vi "Full_LabviewGUI.vi"() -> ()   [LabVIEW 2022 SP3]
doc: "The UDP protocol differs from TCP in that there is no error-checking with the packets of information that are sent, and thus no guarantee whatsoever that an intended recipient will actually receive a given piece of data.\n\nUDP does offer the ability to \"broadcast\" data across a network--simply specify an IP Address of all ones (255.255.255.255) to attempt to broadcast information network-wide. Keep in mind that routers and other network hardware will generally refuse to forward the broadcast beyond certain points, so the extent of the broadcast will in practice be limited."
uses:
  <vilib>/vision/NI_Vision_Development_Module.lvlib
panel:
  out "Sensor 2 (cm)":dbl format="%#_4g"
  out "Sensor 1 (cm)":dbl format="%#_4g"
  in  "?":bool
  in  "Start Automatic Path Following":bool
  out "Image Out":T1(plugin-control)
  in  "Stop (F)":bool caption="Stop Tracking Path"
  out "XY Graph":cluster{"x":sgl, "y":sgl}[](graph)
  in  "Turn left":bool
  in  "Turn right":bool
  in  "Backward":bool
  in  "Forward":bool
  # "User Manual"
  # "1. Manual Control\nTo control the robot using manual mode, hover the cusor on the button and hold on to the click button to move the robot, stop holding the cursor will make the robot stop.\n    The Manual Control panel will be disabled and grayed out when automatic path following is running.\n\n2. Ultrasonic Sensors Data\nThe Ultrasonic Sensors Data panel shows the realtime distance from received from esp32 in the unit of cm.\n\n3. Start Automatic Path Following\nThe Start Automatic Path Following button will open up the terminal and start an anaconda kernel to run the python script that does: obstacle detection, path finding and MPC which does path following. \n    Close windows generated by the python session after its done (recommended)\n\n4. Realtime image and XY graph\nThe two panels shows the location of the robot with its track. Click on the button \"Stop Tracking Path\" to stop plotting on the graph.\n\n5. STOP\nThe stop button terminates all the process and send a final command to terminate the python kernel and stops the robot."
  # "The STOP button will terminate GUI, stop \nthe python kernel and set Jetbot speed to 0"
  # "Manual Control"
  # "Ultrasonic Sensors Data"
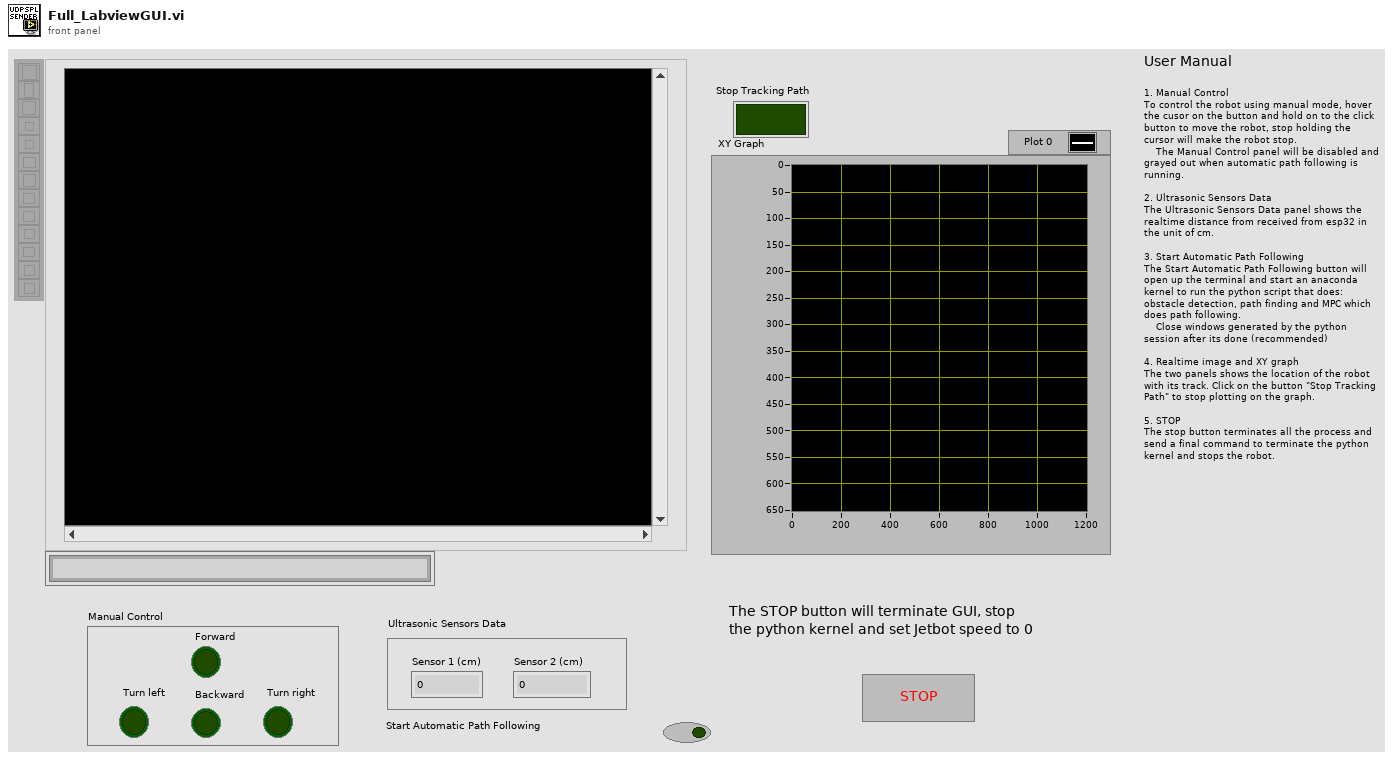
[diagram p1: front panel]
types:
  T1 = typedef "IMAQ Image.ctl" = refnum<image>
  T2 = typedef "Image Type" = u32
  T3 = enum8{"Enabled", "Disabled", "Disabled and Grayed Out"}
  T4 = cluster{"Position":cluster{"x":sgl, "y":sgl}, "Angle":sgl, "Scale":sgl, "Score":sgl, "Bounding Box":cluster{"x":sgl, "y":sgl}[]}[]
  T5 = cluster{"Matches (Pattern Matching 1)[0]":cluster{"Position":cluster{"x":sgl, "y":sgl}, "Angle":sgl, "Scale":sgl, "Score":sgl, "Bounding Box":cluster{"x":sgl, "y":sgl}[]}, "Matches (Pattern Matching 1)[1]":cluster{"Position":cluster{"x":sgl, "y":sgl}, "Angle":sgl, "Scale":sgl, "Score":sgl, "Bounding Box":cluster{"x":sgl, "y":sgl}[]}, "Matches (Pattern Matching 1)[2]":cluster{"Position":cluster{"x":sgl, "y":sgl}, "Angle":sgl, "Scale":sgl, "Score":sgl, "Bounding Box":cluster{"x":sgl, "y":sgl}[]}, "Matches (Pattern Matching 1)[3]":cluster{"Position":cluster{"x":sgl, "y":sgl}, "Angle":sgl, "Scale":sgl, "Score":sgl, "Bounding Box":cluster{"x":sgl, "y":sgl}[]}}
  T6 = cluster{"Bounding Box[0]":cluster{"x":sgl, "y":sgl}, "Bounding Box[1]":cluster{"x":sgl, "y":sgl}, "Bounding Box[2]":cluster{"x":sgl, "y":sgl}, "Bounding Box[3]":cluster{"x":sgl, "y":sgl}}
  T7 = cluster{"[0]":sgl, "[1]":sgl, "[2]":sgl, "[3]":sgl}
  T8 = cluster{"[0]":i32, "[1]":i32, "[2]":i32, "[3]":i32}
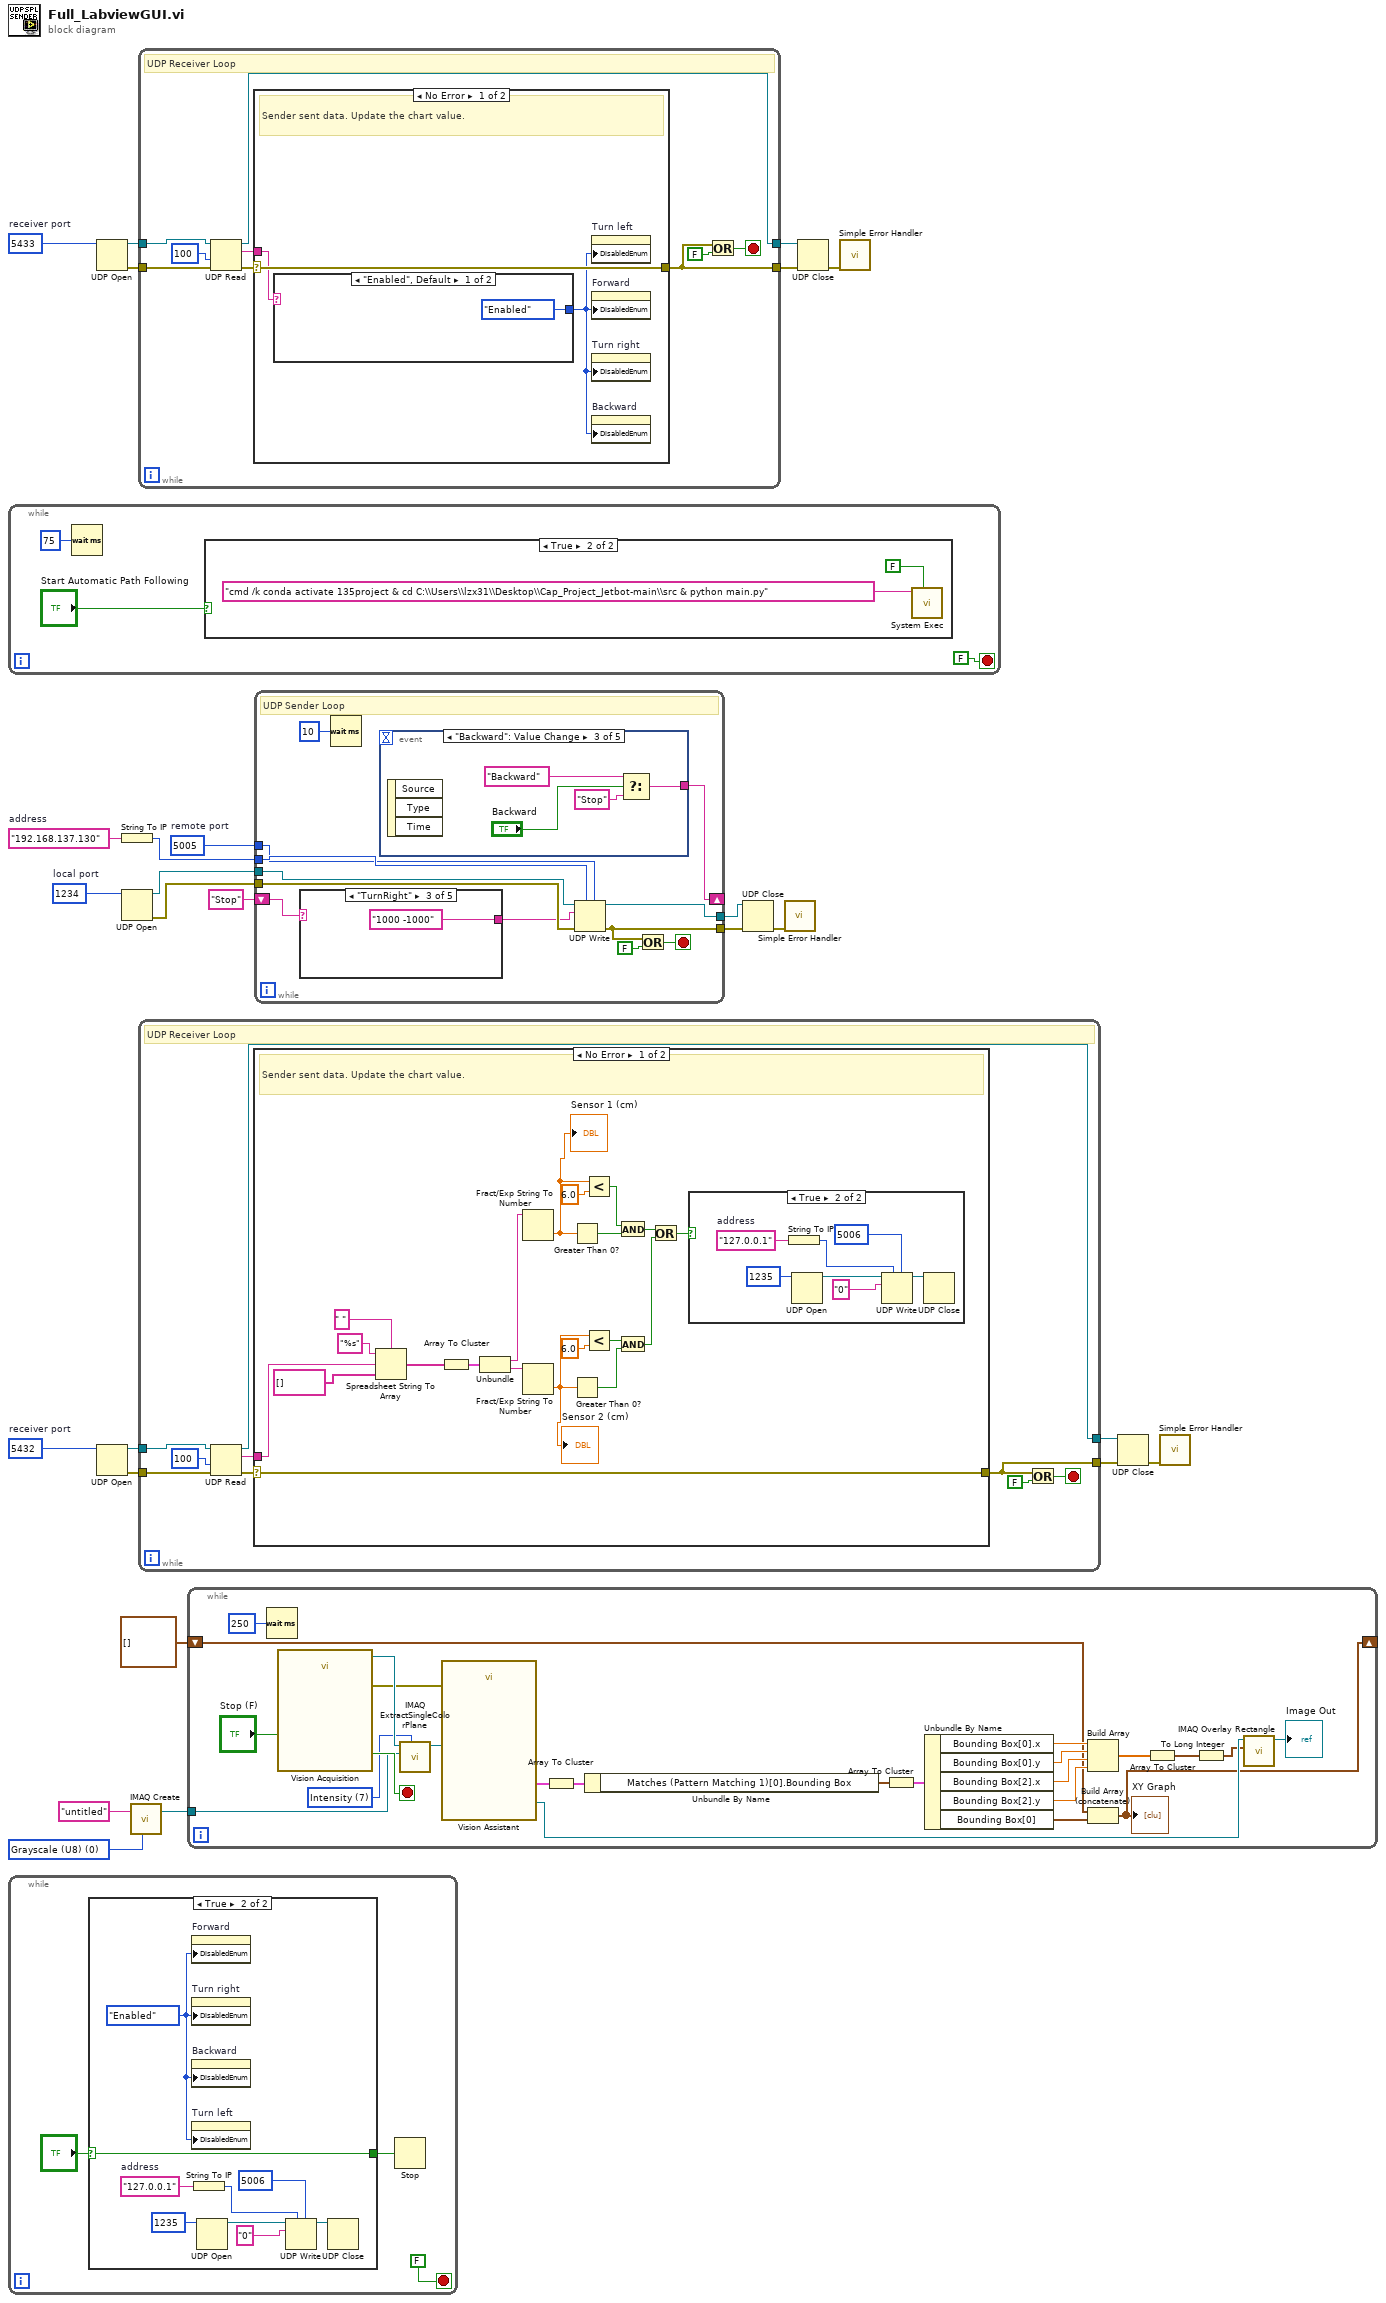
[diagram p0: block diagram]
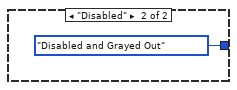
[diagram p2: hidden frame]
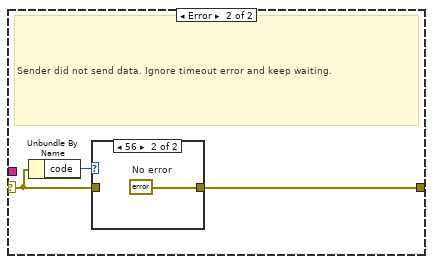
[diagram p3: hidden frame]
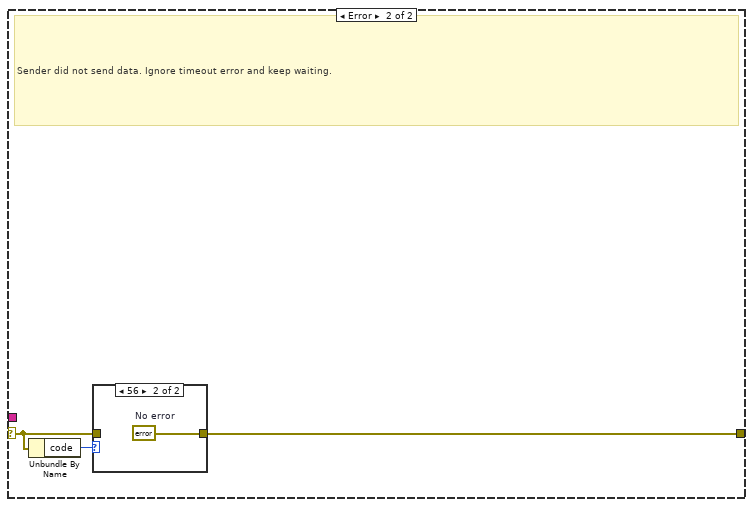
[diagram p8: hidden frame]
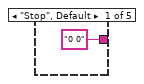
[diagram p10: hidden frame]
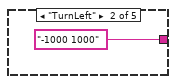
[diagram p11: hidden frame]
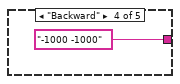
[diagram p12: hidden frame]
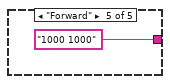
[diagram p13: hidden frame]
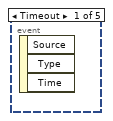
[diagram p14: hidden frame]
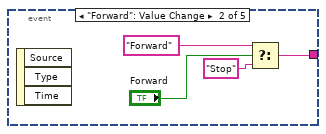
[diagram p15: hidden frame]
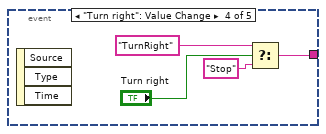
[diagram p16: hidden frame]
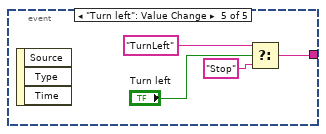
[diagram p17: hidden frame]
diagram:
  w1 = u16 5433  # receiver port
  w9 = T2 0 items=["Grayscale (U8)", "Grayscale (I16)", "Grayscale (SGL)", "Complex (CSG)", "RGB (U32)", "HSL (U32)", "RGB (U64)", "Grayscale (U16)"] ("Image Type")
  w11 = u16 5432  # receiver port
  w18 = u16 5005  # remote port
  w19 = u16 1234  # local port
  w24 = "192.168.137.130"  # address
  n1 = while {
    stop <- FALSE stop-if-true
    n2 = Wait (ms)(milliseconds to wait=u32 75) -> ()  [unwired: 1 out]
    n3 = case shown="True" "Start Automatic Path Following" {
      frame False {
      }
      frame True {
        n4 = call <vilib>:"System Exec.vi"("wait until completion? (T)"=FALSE, "command line"="cmd /k conda activate 135project & cd C:\\Users\\lzx31\\Desktop\\Cap_Project_Jetbot-main\\src & python main.py") -> ()  [unwired: 6 in, 4 out]
      }
    }
  }
  n5 = while {
    stop <- FALSE stop-if-true
    n6 = case shown="True" "?" {
      selector: "?" -> [w35 w37]
      tunnel: [w35 w37] -> w33
      frame False {
      }
      frame True {
        w36 = T3."Enabled" ("Disabled")
        w43 = "127.0.0.1"  # address
        n7 = property on="Forward" class="Bool (strict)"("DisabledEnum"=w36) -> ()  [unwired: 2 in, 2 out]
        n8 = property on="Turn right" class="Bool (strict)"("DisabledEnum"=w36) -> ()  [unwired: 2 in, 2 out]
        n9 = property on="Backward" class="Bool (strict)"("DisabledEnum"=w36) -> ()  [unwired: 2 in, 2 out]
        n10 = property on="Turn left" class="Bool (strict)"("DisabledEnum"=w36) -> ()  [unwired: 2 in, 2 out]
        n11 = String To IP(1:w43) -> (0:w42:u32)
        n12 = UDP Open(11:u16 1235 ("port")) -> (port=w41:refnum<k16>)  [unwired: 4 in, 2 out]
        n13 = UDP Write(address=w42, port or service name=u16 5006, connection ID=w41, data in="0") -> (3:w39:refnum<k16>)  [unwired: 2 in, 1 out]
        n14 = UDP Close(connection ID=w39) -> ()  [unwired: 1 in, 2 out]
      }
    }
    n15 = Stop(stop? (T)=w33) -> ()
  }
  n16 = UDP Open(11:w1) -> (port=w2:refnum<k16>, 0:w3:errorcluster)  [unwired: 4 in, 1 out]
  n17 = UDP Open(11:w11) -> (port=w12:refnum<k16>, 0:w13:errorcluster)  [unwired: 4 in, 1 out]
  n18 = String To IP(1:w24) -> (0:w22:u32)
  n19 = UDP Open(11:w19) -> (port=w21:refnum<k16>, 0:w20:errorcluster)  [unwired: 4 in, 1 out]
  n20 = call "IMAQ Create"("Image Name"="untitled", "Image Type"=w9) -> ("New Image"=w8:T1)  [unwired: 3 in, 1 out]
  n21 = while {
    tunnel: w2 -> [w53]
    tunnel: [w45] -> w6
    tunnel: w3 -> [w50]
    tunnel: [w46] -> w4
    stop <- w51 stop-if-true
    # "UDP Receiver Loop"
    n22 = UDP Read(connection ID=w53, timeout ms (25000)=100, 8:w50) -> (data out=w48:string, error out=w47:errorcluster, 3:w45:refnum<k16>)  [unwired: 3 out]
    n23 = case shown="No Error" w47 {
      selector: w47 -> [w56 w60]
      tunnel: w48 -> [w55 _]
      tunnel: [w56 w59] -> w46
      frame No Error {
        # "Sender sent data. Update the chart value."
        n24 = case shown="\"Enabled\", Default" w55 {
          tunnel: [T3."Enabled" ("Disabled") T3."Disabled and Grayed Out" ("Disabled")] -> w54
          frame "Enabled", Default {
          }
          frame "Disabled" {
          }
        }
        n25 = property on="Turn left" class="Bool (strict)"("DisabledEnum"=w54) -> ()  [unwired: 2 in, 2 out]
        n26 = property on="Forward" class="Bool (strict)"("DisabledEnum"=w54) -> ()  [unwired: 2 in, 2 out]
        n27 = property on="Turn right" class="Bool (strict)"("DisabledEnum"=w54) -> ()  [unwired: 2 in, 2 out]
        n28 = property on="Backward" class="Bool (strict)"("DisabledEnum"=w54) -> ()  [unwired: 2 in, 2 out]
      }
      frame Error {
        # "Sender did not send data. Ignore timeout error and keep waiting."
        n29 = Unbundle By Name(w60) -> ("code"=w61:i32)
        n30 = case shown="56" w61 {
          tunnel: w60 -> [w62 _]
          tunnel: [w62 w63] -> w59
          frame Default {
          }
          frame 56 {
            w63 = errorcluster {"status"=FALSE, "code"=0, "source"=""}  # No error
          }
        }
      }
    }
    n31 = Or(x=w46, y=FALSE ("Stop 2")) -> (x .or. y?=w51:bool)
  }
  n32 = while {
    tunnel: w12 -> [w72]
    tunnel: [w64] -> w16
    tunnel: w13 -> [w69]
    tunnel: [w65] -> w14
    stop <- w70 stop-if-true
    # "UDP Receiver Loop"
    n33 = UDP Read(connection ID=w72, timeout ms (25000)=100, 8:w69) -> (data out=w67:string, error out=w66:errorcluster, 3:w64:refnum<k16>)  [unwired: 3 out]
    n34 = case shown="No Error" w66 {
      selector: w66 -> [w92 w101]
      tunnel: w67 -> [w80 _]
      tunnel: [w92 w100] -> w65
      frame No Error {
        # "Sender sent data. Update the chart value."
        n35 = Spreadsheet String To Array(delimiter (Tab)=" ", format string="%s", spreadsheet string=w80, array type (2D Dbl)=string[] []) -> (array=w88:string[])
        n36 = Array To Cluster(array=w88) -> (cluster=w87:cluster{"[0]":string, "[1]":string})
        n37 = Unbundle(w87) -> ("[0]"=w76:string, "[1]"=w75:string)
        n38 = Fract/Exp String To Number(string=w76) -> (number=w74:dbl)  [unwired: 3 in, 1 out]
        "Sensor 1 (cm)" <- w74
        n39 = Fract/Exp String To Number(string=w75) -> (number=w73:dbl)  [unwired: 3 in, 1 out]
        "Sensor 2 (cm)" <- w73
        n40 = Greater Than 0?(x=w74) -> (x > 0?=w86:bool)
        n41 = Greater Than 0?(x=w73) -> (x > 0?=w84:bool)
        n42 = Less?(x=w74, y=6.0 ("x")) -> (x < y?=w85:bool)
        n43 = Less?(x=w73, y=6.0) -> (x < y?=w83:bool)
        n44 = And(x=w85, y=w86) -> (x .and. y?=w82:bool)
        n45 = And(x=w83, y=w84) -> (x .and. y?=w81:bool)
        n46 = Or(x=w82, y=w81) -> (x .or. y?=w79:bool)
        n47 = case shown="True" w79 {
          frame False {
          }
          frame True {
            w98 = "127.0.0.1"  # address
            n48 = String To IP(1:w98) -> (0:w97:u32)
            n49 = UDP Open(11:u16 1235 ("port")) -> (port=w96:refnum<k16>)  [unwired: 4 in, 2 out]
            n50 = UDP Write(address=w97, port or service name=u16 5006, connection ID=w96, data in="0") -> (3:w94:refnum<k16>)  [unwired: 2 in, 1 out]
            n51 = UDP Close(connection ID=w94) -> ()  [unwired: 1 in, 2 out]
          }
        }
      }
      frame Error {
        # "Sender did not send data. Ignore timeout error and keep waiting."
        n52 = Unbundle By Name(w101) -> ("code"=w102:i32)
        n53 = case shown="56" w102 {
          tunnel: w101 -> [w103 _]
          tunnel: [w103 w104] -> w100
          frame Default {
          }
          frame 56 {
            w104 = errorcluster {"status"=FALSE, "code"=0, "source"=""}  # No error
          }
        }
      }
    }
    n54 = Or(x=w65, y=FALSE ("Stop 2")) -> (x .or. y?=w70:bool)
  }
  n55 = while {
    tunnel: w8 -> [w126]
    shift-right: [w107] -> _
    shift-left: cluster{"x":sgl, "y":sgl}[] [] -> [w106]
    stop <- w127 stop-if-true
    w124 = 7 items=["Red", "Green", "Blue", "Hue", "Saturation", "Luminance", "Value", "Intensity"] ("Color Plane")
    n56 = Wait (ms)(milliseconds to wait=u32 250 ("millisecond timer value")) -> ()  [unwired: 1 out]
    n57 = call "Vision Acquisition"("Stop (F)"="Stop (F)") -> ("Image Out"=w125:T1, "Stopped"=w127:bool, "error out"=w122:errorcluster)  [unwired: 24 in]
    n58 = call "IMAQ ExtractSingleColorPlane"("Color Plane"=w124, "Image Dst"=w126, "Image Src"=w125) -> ("Image Dst Out"=w123:T1)  [unwired: 7 in, 1 out]
    n59 = call "Vision Assistant"("Image In"=w123, "error in"=w122) -> ("Image Out"=w113:T1, "Matches (Pattern Matching 1)"=w121:T4)  [unwired: 23 in, 1 out]
    n60 = Array To Cluster(array=w121) -> (cluster=w120:T5)
    n61 = Unbundle By Name(w120) -> ("Matches (Pattern Matching 1)[0].Bounding Box"=w119:cluster{"x":sgl, "y":sgl}[])
    n62 = Array To Cluster(array=w119) -> (cluster=w118:T6)
    n63 = Unbundle By Name(w118) -> ("Bounding Box[0].x"=w117:sgl, "Bounding Box[0].y"=w116:sgl, "Bounding Box[2].x"=w115:sgl, "Bounding Box[2].y"=w114:sgl, "Bounding Box[0]"=w108:cluster{"x":sgl, "y":sgl})
    n64 = Build Array(w117, w116, w115, w114) -> (w109:sgl[])
    n65 = Build Array (concatenate)(w106, w108) -> (w107:cluster{"x":sgl, "y":sgl}[])
    "XY Graph" <- w107
    n66 = Array To Cluster(array=w109) -> (cluster=w111:T7)
    n67 = To Long Integer(number=w111) -> (32bit integer=w110:T8)
    n68 = call "IMAQ Overlay Rectangle"("Rectangle"=w110, "Image"=w113) -> ("Image Out"=→"Image Out":T1)  [unwired: 8 in, 1 out]
  }
  n69 = while {
    tunnel: [w135] -> w25
    tunnel: w21 -> [w140]
    tunnel: w20 -> [w139]
    tunnel: [w136] -> w26
    tunnel: w22 -> [w134]
    tunnel: w18 -> [w132]
    shift-right: [w130] -> _
    shift-left: "Stop" -> [w131]
    stop <- w138 stop-if-true
    # "UDP Sender Loop"
    n70 = case shown="\"TurnRight\"" w131 {
      tunnel: ["0 0" "-1000 1000" "1000 -1000" "-1000 -1000" "1000 1000"] -> w129
      frame "Stop", Default {
      }
      frame "TurnLeft" {
      }
      frame "TurnRight" {
      }
      frame "Backward" {
      }
      frame "Forward" {
      }
    }
    n71 = Wait (ms)(milliseconds to wait=u32 10) -> ()  [unwired: 1 out]
    n72 = event shown="[2] \"Backward\": Value Change" {
      selector: _ -> [_ _ _ _ _]
      dyn-events: _ -> [_ _ _ _ _]
      timeout: _ -> [_ _ _ _ _]
      tunnel: [_ w148 w150 w154 w158] -> w130
      event Timeout {
        n73 = event-data() -> ()  [unwired: 1 in, 3 out]
      }
      event "Forward": Value Change {
        n74 = event-data() -> ()  [unwired: 1 in, 3 out]
        n75 = Select(t="Forward", s="Forward", f="Stop") -> (s? t:f=w148:string)
      }
      event "Backward": Value Change {
        n76 = event-data() -> ()  [unwired: 1 in, 3 out]
        n77 = Select(t="Backward", s="Backward", f="Stop") -> (s? t:f=w150:string)
      }
      event "Turn right": Value Change {
        n78 = event-data() -> ()  [unwired: 1 in, 3 out]
        n79 = Select(t="TurnRight", s="Turn right", f="Stop") -> (s? t:f=w154:string)
      }
      event "Turn left": Value Change {
        n80 = event-data() -> ()  [unwired: 1 in, 3 out]
        n81 = Select(t="TurnLeft", s="Turn left", f="Stop") -> (s? t:f=w158:string)
      }
    }
    n82 = UDP Write(address=w134, port or service name=w132, connection ID=w140, data in=w129, 8:w139) -> (error out=w135:errorcluster, 3:w136:refnum<k16>)  [unwired: 1 in]
    n83 = Or(x=w135, y=FALSE ("Stop")) -> (x .or. y?=w138:bool)
  }
  n84 = UDP Close(connection ID=w26, 8:w25) -> (error out=w23:errorcluster)  [unwired: 1 out]
  n85 = call <vilib>:"Simple Error Handler.vi"("error in (no error)"=w23) -> ()  [unwired: 4 in, 5 out]
  n86 = UDP Close(connection ID=w6, 8:w4) -> (error out=w5:errorcluster)  [unwired: 1 out]
  n87 = call <vilib>:"Simple Error Handler.vi"("error in (no error)"=w5) -> ()  [unwired: 1 in, 8 out]
  n88 = UDP Close(connection ID=w16, 8:w14) -> (error out=w15:errorcluster)  [unwired: 1 out]
  n89 = call <vilib>:"Simple Error Handler.vi"("error in (no error)"=w15) -> ()  [unwired: 1 in, 8 out]
